vi "Report_Data.vi"(2 "Error In":errorcluster, 3 "Values":string[](array[string])) -> (0 "Error Out":errorcluster)   [LabVIEW 2019]
uses:
  Global Variables/Global_Variables.vi
  <vilib>/Utility/file.llb/Write Delimited Spreadsheet (string).vi
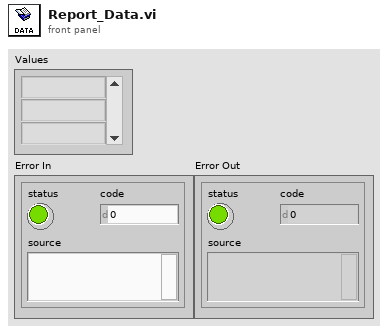
[diagram p1: front panel]
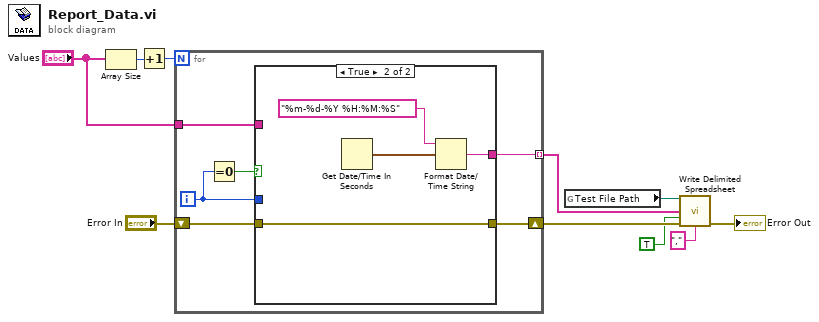
[diagram p0: block diagram]
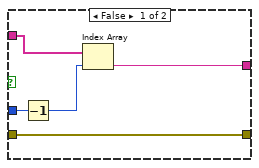
[diagram p2: hidden frame]
diagram:
  n1 = Array Size(array="Values") -> (size(s)=w4:i32)
  n2 = Increment(x=w4) -> (x+1=w5:i32)
  n3 = for {
    N: w5 -> [_]
    shift-right: [w13] -> w9
    shift-left: "Error In" -> [w14]
    tunnel: [w12] -> w1 mode=indexing
    tunnel: "Values" -> [w11]
    i -> [w15]
    n4 = Equal To 0?(x=w15) -> (x = 0?=w16:bool)
    n5 = case shown="True" w16 {
      tunnel: w14 -> [w21 w25]
      tunnel: [w21 w25] -> w13
      tunnel: [w17 w22] -> w12
      tunnel: w15 -> [w20 _]
      tunnel: w11 -> [w19 _]
      frame False {
        n6 = Decrement(x=w20) -> (x-1=w18:i32)
        n7 = Index Array(array=w19, index=w18) -> (element=w17:string)
      }
      frame True {
        n8 = Get Date/Time In Seconds() -> (seconds since 1Jan1904=w24:timestamp)
        n9 = Format Date/Time String(time format string (%c)="%m-%d-%Y %H:%M:%S", seconds (now)=w24) -> (date/time string=w22:string)  [unwired: 1 in]
      }
    }
  }
  n10 = global read "Global_Variables.vi" "Test File Path"() -> (w7:path)
  n11 = call-poly <vilib>:"Write Delimited Spreadsheet.vi"("file path (dialog if empty)"=w7, "1D data"=w1, "append to file? (new file:F)"=TRUE, "error in (no error)"=w9, "delimiter (\\t)"="," ("delimiter (\\t)")) -> ("error out"=→"Error Out":errorcluster)  [unwired: 9 in, 1 out]
